vi "Variant to DBL or DBL Array.vi"(8 "error in (no error)":errorcluster, 11 "value":variant) -> (0 "error out":errorcluster, 3 "Array":dbl[](array[numeric]))   [LabVIEW 2016, in "LVtoITX.lvclass"]
uses:
  LVtoITX.lvclass
  <vilib>/Utility/Data Type/NI_Data Type.lvlib
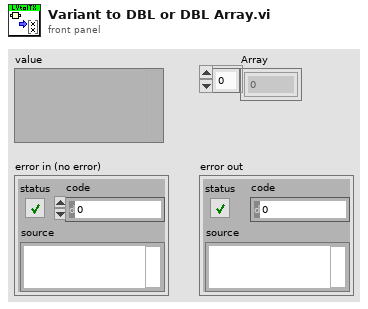
[diagram p1: front panel]
types:
  T1 = typedef "NI_Data Type.lvlib/Data Type.ctl" = enum8{"Invalid Type", "Void", "I8", "I16", "I32", "I64", "U8", "U16", "U32", "U64", "Single Float", "Double Float", "Extended Float", "Single Complex", "Double Complex", "Extended Complex", "Enum U8", "Enum U16", "Enum U32", "Enum U64", "Single Float With Unit", "Double Float With Unit", "Extended Float With Unit", "Single Complex with Unit", "Double Complex with Unit", "Extended Complex with Unit", "Boolean", "String", "Path", "Picture", "Tag", "Array", "Cluster", "Variant", "LV Variant", "Waveform", "Timestamp", "Digital Waveform", "Digital Data", "ExpressData", "Refnum", "External Data", "VI", "Poly VI", "LabVIEW Class Instance", "Fixed Point"}
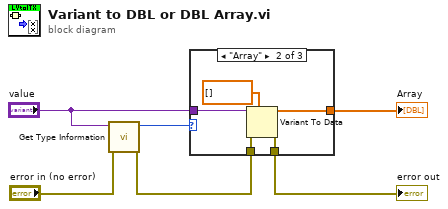
[diagram p0: block diagram]
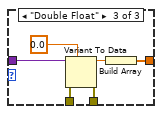
[diagram p3: hidden frame]
diagram:
  n1 = call <vilib>:"Get Type Information.vi"("error in (no error)"="error in (no error)", "Variant"="value") -> ("error out"=w5:errorcluster, "Type"=w6:T1)  [unwired: 5 in, 3 out]
  n2 = case shown="\"Array\"" w6 {
    tunnel: [w7 w11 w18] -> w2
    tunnel: [_ w10 w13] -> w3
    tunnel: "value" -> [_ w9 w16]
    tunnel: w5 -> [w7 w8 w15]
    frame Default {
    }
    frame "Array" {
      n3 = Variant To Data(error in=w8, type=dbl[] [], Variant=w9) -> (data=w10:dbl[], error out=w11:errorcluster)
    }
    frame "Double Float" {
      n4 = Variant To Data(error in=w15, type=0.0, Variant=w16) -> (data=w17:dbl, error out=w18:errorcluster)
      n5 = Build Array(w17) -> (w13:dbl[])
    }
  }
  "Array" <- w3
  "error out" <- w2
